vi "Error Scan Information.vi"(2 "Error Code":u8 format="%.0x", 8 "error in (no error)":errorcluster, 10 "Data Valid":bool, 11 "Siemens Ctr":T1) -> (0 "error out":errorcluster {"code" format="%.0x"}, 3 "Siemens Ctr out":T1)   [LabVIEW 2014, in "Simatic S7.lvlib"]
uses:
  Simatic S7.lvlib
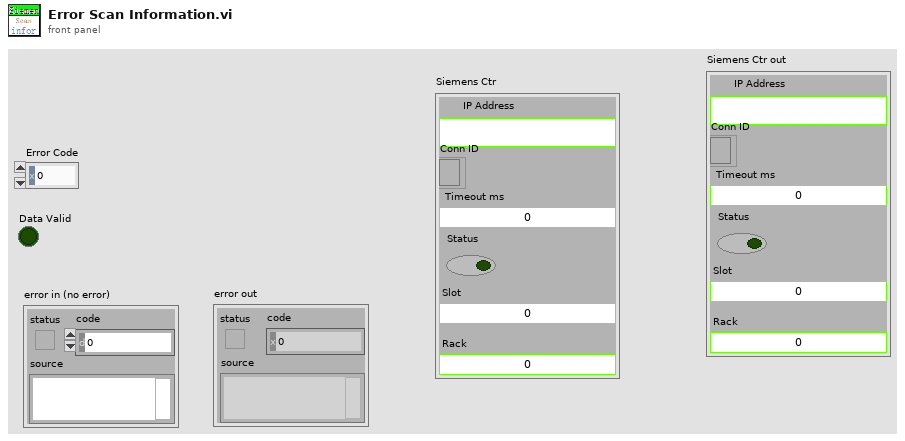
[diagram p1: front panel]
types:
  T1 = typedef "Simatic S7.lvlib/Siemens Ref.ctl" = cluster{"IP Address ":string, "Conn ID":refnum<k5>, "Timeout ms":i32, "Status":bool, "Slot":u16, "Rack":u16}
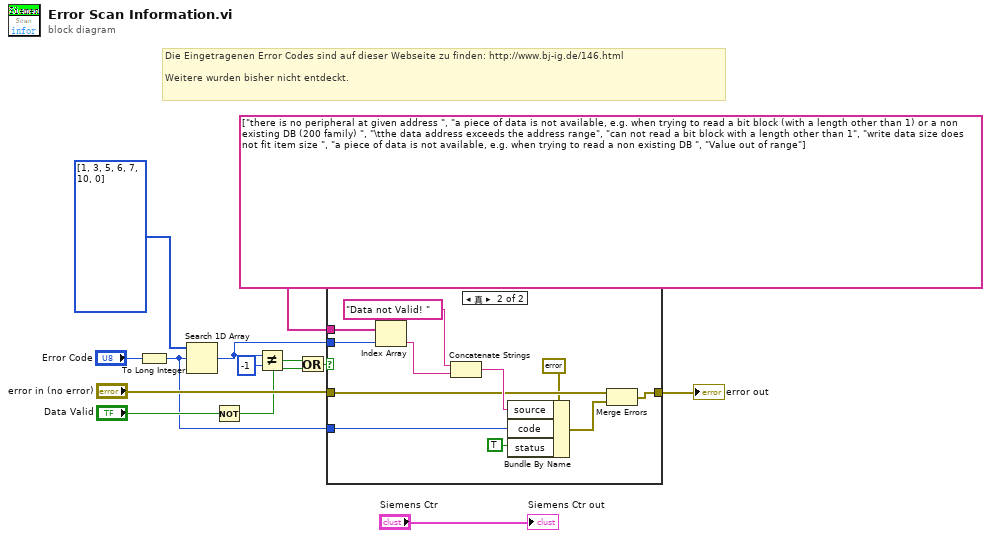
[diagram p0: block diagram]
diagram:
  # "Die Eingetragenen Error Codes sind auf dieser Webseite zu finden: http://www.bj-ig.de/146.html\n\nWeitere wurden bisher nicht entdeckt."
  n1 = To Long Integer(number="Error Code") -> (32bit integer=w3:i32)
  n2 = Search 1D Array(1D array=i32[] [1, 3, 5, 6, 7, 10, 0] ("[user-defined codes]"), element=w3) -> (index of element=w9:i32)  [unwired: 1 in]
  n3 = Not(x="Data Valid") -> (.not. x?=w2:bool)
  n4 = Not Equal?(x=w9, y=-1) -> (x != y?=w5:bool)
  n5 = Or(x=w5, y=w2) -> (x .or. y?=w4:bool)
  n6 = case shown="真" w4 {
    tunnel: string[] ["there is no peripheral at given address ", "a piece of data is not available, e.g. when trying to read a bit block (with a length other than 1) or a non existing DB (200 family) ", "\tthe data address exceeds the address range", "can not read a bit block with a length other than 1", "write data size does not fit item size ", "a piece of data is not available, e.g. when trying to read a non existing DB ", "Value out of range"] ("[user-defined descriptions]") -> [_ w25]
    tunnel: w9 -> [_ w24]
    tunnel: "error in (no error)" -> [w14 w18]
    tunnel: [w14 w15] -> w7
    tunnel: w3 -> [_ w22]
    frame False {
    }
    frame True {
      n7 = Index Array(array=w25, index=w24) -> (element=w21:string)
      n8 = Concatenate Strings("Data not Valid! " ("source"), w21) -> (w19:string)
      n9 = Bundle By Name(cluster=errorcluster {"status"=FALSE, "code"=0, "source"=""} ("error out"), "source"=w19, "code"=w22, "status"=TRUE) -> (w16:errorcluster)
      n10 = Merge Errors(w18, w16) -> (w15:errorcluster)
    }
  }
  "error out" <- w7
  "Siemens Ctr out" <- "Siemens Ctr"
